vi "Image_resize.vi"(9 "String":string, 10 "stripped path":path, 11 "Picture in":refnum<vi>) -> (3 "2D Picture":picture)   [LabVIEW 2015]
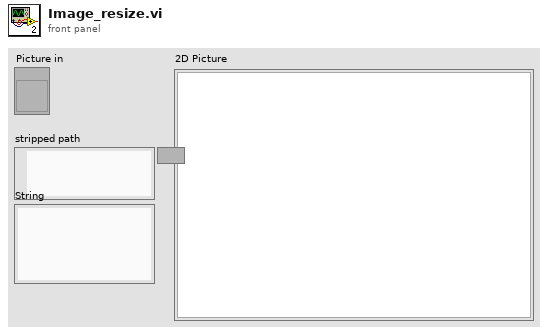
[diagram p1: front panel]
types:
  T1 = typedef "LVBoundsTypeDef.ctl" = cluster{"Width":u32, "Height":u32}
  T2 = typedef "imagedata.ctl" = cluster{"image type":i32, "image depth":i32, "image":u8[], "mask":u8[], "colors":u32[], "Rectangle":cluster{"left":i16, "top":i16, "right":i16, "bottom":i16}}
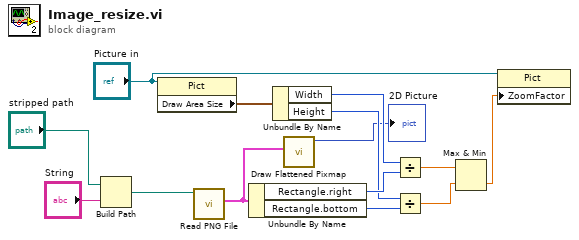
[diagram p0: block diagram]
diagram:
  n1 = Build Path(base path="stripped path", name or relative path="String") -> (appended path=w5:path)
  n2 = property on="Property Node" class="Pict"(reference="Picture in") -> ("Draw Area Size"=w7:T1)  [unwired: 1 in, 2 out]
  n3 = call <vilib>:"Read PNG File.vi"("path to PNG file"=w5) -> ("image data"=w6:T2)  [unwired: 8 in, 2 out]
  n4 = Unbundle By Name(w6) -> ("Rectangle.right"=w10:i16, "Rectangle.bottom"=w11:i16)
  n5 = Unbundle By Name(w7) -> ("Width"=w8:u32, "Height"=w9:u32)
  n6 = call <vilib>:"Draw Flattened Pixmap.vi"("image data"=w6) -> ("new picture"=→"2D Picture":picture)  [unwired: 8 in]
  n7 = Divide(x=w8, y=w10) -> (x/y=w12:dbl)
  n8 = Divide(x=w9, y=w11) -> (x/y=w13:dbl)
  n9 = Max & Min(x=w12, y=w13) -> (min(x,y)=w14:dbl)  [unwired: 1 out]
  n10 = property on="Property Node" class="Pict"(reference="Picture in", "ZoomFactor"=w14) -> ()  [unwired: 1 in, 2 out]
